vi "Tick Duration (with error).vi"(8 "error in (no error)":errorcluster, 10 "tick count before":u32) -> (0 "error out":errorcluster, 2 "tick count after [ms]":u32, 3 "duration [ms]":u32)   [LabVIEW 2016]
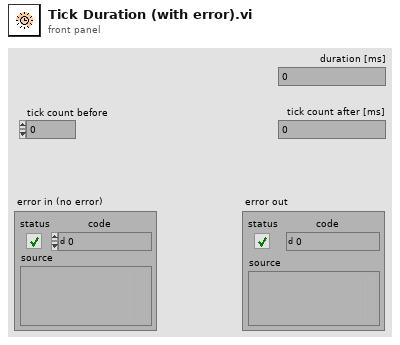
[diagram p1: front panel]
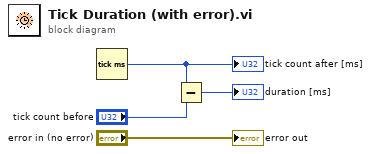
[diagram p0: block diagram]
diagram:
  n1 = Tick Count (ms)() -> (millisecond timer value=w1:u32)
  "tick count after [ms]" <- w1
  n2 = Subtract(x=w1, y="tick count before") -> (x-y=→"duration [ms]":u32)
  "error out" <- "error in (no error)"
